vi "ADC Offset Gain_test.vi"(8 "error in (no error)":errorcluster, 9 "Sequence parameters":string[][](array[string])=[["Min limit", "Max limit", "Register sheet file", "Register Sheet"], ["", "", "CC2600.xls", "TX_BLE;Trim"], ["Reg write (addr;value)", "Operating frequency [Hz]", "", ""], ["NA", "2.44G", "", ""]], 10 "Run type":i32, 11 "Method parameters":T3={"Dev"={"Do not disturb DUT"=FALSE, "XOSC"=32000000.0, "Board type"="", "EM"="", "Configure tempboard"=TRUE, "Device specific info"=[], "Generic Object"=refnum}, "Method"={"Run type"=1, "Test name"="Current LPM2 4", "Comment"="", "Results folder"="", "AFC"=enum."Off", "Method name"="Current LPM2 4", "Method results"={"Excel brief report"=FALSE, "Spotfire report"=FALSE, "Starfish report"=FALSE}, "Operator"="", "Reference time"=timestamp(0 s since 1904-01-01), "AFC delay"=0.0, "Initialization"=enum."Enabled", "MD5 Sum"="", "HW addon board"=enum."None", "AFC Regsheet"="", "AFC Regfile"=path "", "dummy"=0.0}, "Inst"={"Instr"={"PS1"={"Name"="", "GPIB address"="", "VISA session"=""}, "PS2"={"Name"="", "GPIB address"="", "VISA session"=""}, "TC1"={"Name"="", "GPIB address"="", "VISA session"=""}, "TC2"={"Name"="", "GPIB address"="", "VISA session"=""}, "SA1"={"Name"="", "GPIB address"="", "VISA session"=""}, "SA2"={"Name"="", "GPIB address"="", "VISA session"=""}, "SG1"={"Name"="", "GPIB address"="", "VISA session"=""}, "SG2"={"Name"="", "GPIB address"="", "VISA session"=""}, "SG3"={"Name"="", "GPIB address"="", "VISA session"=""}, "MI1"={"Name"="", "GPIB address"="", "VISA session"=""}, "MI2"={"Name"="", "GPIB address"="", "VISA session"=""}, "SW SA"={"Name"="", "Controller addr"=""}, "SW SG"={"Name"="", "Controller addr"=""}, "MI3"={"Name"="", "GPIB address"="", "VISA session"=""}}, "Switchbox"={"RF Path"=0, "Cal compensation"=enum."TX", "Switchbox gain mode"="", "State"=enum."TX"}, "Instr to control (i.e. SA1)"="Default", "Intrument info string"=""}, "Sequence parameters"=[["Weight", "Min Limit", "Max Limit", "Register Sheet", "", "", "", "", "", "", "", "", ""], ["Vital", "", "1", "LPM2", "", "", "", "", "", "", "", "", ""], ["Resolution", "Reg write (addr;value)", "Chip mode", "Range", "", "", "", "", "", "", "", "", ""], ["u", "NA", "", "auto", "", "", "", "", "", "", "", "", ""]], "Cond"={"Temp logged"=25.0, "VDD1_PS1_6V"=-999.0, "VDD2_PS1_25V"=-999.0, "VDD4_PS2_25V"=-999.0, "VDD3_PS2_6V"=-999.0}, "Meas config"={"X-axis inner loop index"=32000000, "Y-axis outer loop index"=32000000, "X-axis"=[], "Y-axis"=[], "X-axis array req size"=32000000, "Y-axis array req size"=32000000, "Param description"=[], "Use meas clust for reporting"=FALSE, "Parameter index (page)"=0, "X-axis name"="", "Y-axis name"=""}} {"Cond"."VDD3_PS2_6V" format="%.3f"; "Cond"."VDD4_PS2_25V" format="%.3f"; "Cond"."VDD2_PS1_25V" format="%.3f"; "Cond"."VDD1_PS1_6V" format="%.3f"; "Method"."dummy" format="%.1p"; "Method"."AFC delay" format="%.1p"; "Dev"."XOSC" format="%.3p"}) -> (0 "error out":errorcluster, 1 "End method error":T2, 2 "Short Results":string[](array[string])=["0.00", "0.00", "0.00", "0.00"], 3 "Result summary":string[][](array[string])=[["Critical", "Output Power@2405 MHz", "-3", "4", "dBm"], ["Critical", "Output Power@2410 MHz", "-3", "4", "dBm"]])   [LabVIEW 2019]
doc: "[AutoDocStart]Performs crystal accuracy measurements. Measures the offset from ideal frequency. Primarily used for tuning XOSC capacitors and verifying XOSC trims.\n\nSweeping parameters: operating frequency, OSC override value and VDDR level\n\nResults: Offset frequency in ppm[AutoDocEnd]"
uses:
  User Lib/Utilities/Cluster definitions/Method input.ctl
  User Lib/Utilities/Cluster definitions/Device specific info.ctl
  User Lib/Utilities/Controls/Automatic Frequency Compensation types.ctl
  User Lib/Utilities/Controls/Method Reports.ctl
  User Lib/Utilities/Cluster definitions/Method Initialization.ctl
  User Lib/Utilities/Controls/HW addon boards.ctl
  User Lib/Utilities/Cluster definitions/Instr clust.ctl
  User Lib/Utilities/Switchbox control/SwitchBox_State._ENUMctl.ctl
  User Lib/Utilities/Cluster definitions/End method error cluster.ctl
  User Lib/Utilities/Cluster definitions/DUT vdd control.ctl
  User Lib/Utilities/Cluster definitions/DUT VDD4.ctl
  User Lib/Utilities/Cluster definitions/DUT VDD3.ctl
  User Lib/Utilities/Cluster definitions/DUT VDD2.ctl
  User Lib/Utilities/Cluster definitions/DUT VDD1.ctl
  User Lib/Generic chip methods/Classes/Generic_EM/Chameleon/Loki/Loki.lvclass
  <vilib>/Utility/error.llb/Clear Errors.vi
  User Lib/Generic chip methods/Classes/Generic_EM/Chameleon/65nm.lvclass
  C:/Kharon/User Lib/Generic chip methods/Classes/Generic_EM/Generic_EM/Generic_EM.lvclass
  User Lib/Generic chip methods/board_to_chip_type.vi
  User Lib/Generic chip methods/Classes/Get_Class_init.vi
  User Lib/Generic chip methods/Classes/Generic_EM/Generic_EM/Generic_EM.lvclass
  <vilib>/Analysis/NI_AALPro.lvlib
panel:
  out "x/y":dbl
  in  "Tab Control":T1(tab)
  out "Output Response [All DUTs]":u32[][](array[numeric])
  out "Measure Codes":dbl[](array[numeric])
  out "intercept":dbl
  out "slope":dbl
  out "Offset Error (mV)":dbl
  out "Gain Error (LSB)":dbl
  # "°C"
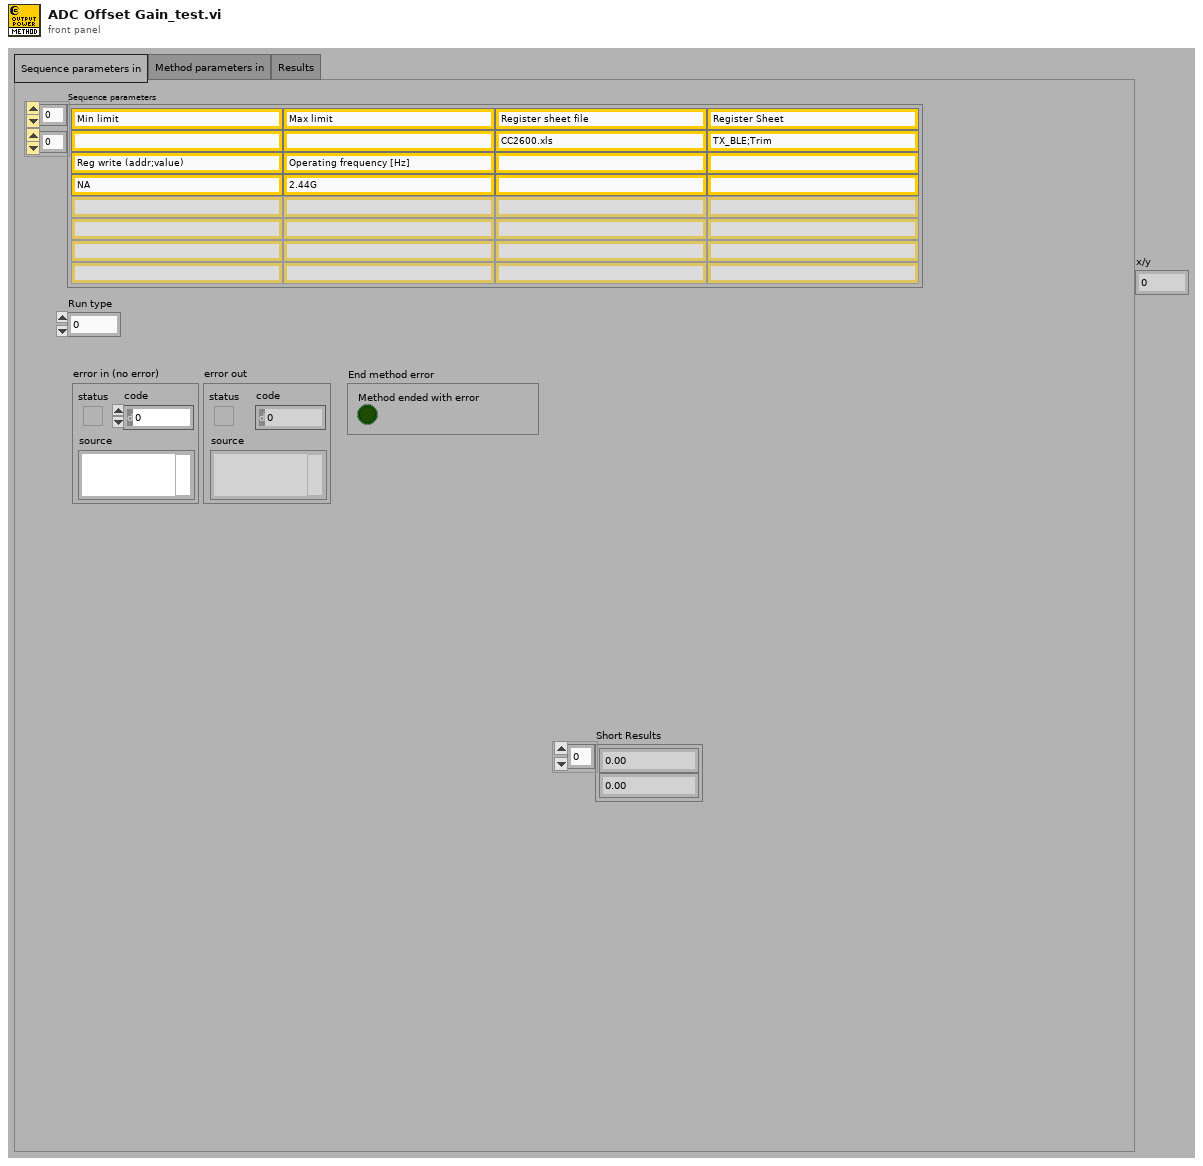
[diagram p1: front panel]
types:
  T1 = enum32{"Sequence parameters in", "Method parameters in", "Results"}
  T2 = typedef "End method error cluster.ctl" = cluster{"Method ended with error":bool}
  T3 = typedef "Method input.ctl" = cluster{"Dev":cluster{"Do not disturb DUT":bool, "XOSC":dbl, "Board type":string, "EM":string, "Configure tempboard":bool, "Device specific info":T4[], "Generic Object":refnum<class>}, "Method":cluster{"Run type":i32, "Test name":string, "Comment":string, "Results folder":string, "AFC":T5, "Method name":string, "Method results":T6, "Operator":string, "Reference time":timestamp, "AFC delay":dbl, "Initialization":T7, "MD5 Sum":string, "HW addon board":T8, "AFC Regsheet":string, "AFC Regfile":path, "dummy":dbl}, "Inst":T9, "Sequence parameters":string[][], "Cond":cluster{"Temp logged":dbl, "VDD1_PS1_6V":dbl, "VDD2_PS1_25V":dbl, "VDD4_PS2_25V":dbl, "VDD3_PS2_6V":dbl}, "Meas config":cluster{"X-axis inner loop index":i32, "Y-axis outer loop index":i32, "X-axis":string[], "Y-axis":string[], "X-axis array req size":i32, "Y-axis array req size":i32, "Param description":string[][], "Use meas clust for reporting":bool, "Parameter index (page)":i32, "X-axis name":string, "Y-axis name":string}}
  T4 = typedef "Device specific info.ctl" = cluster{"EM number":u8, "IP address":string, "Enabled":bool, "Slot no":u8, "RF path":u8, "EM name":string, "Wafer info":string, "AFC frequency ppm":dbl, "Register writes":string[][], "Meas data":string[][][], "Device comment":string}
  T5 = typedef "Automatic Frequency Compensation types.ctl" = enum16{"Off", "Compensate Instrument frequency", "Compensate DUT frequency", "Predictive - Compensate Instrument frequency", "Predictive - Compensate DUT frequency", "Do not skip re-init - Compensate Instrument frequency", "Do not skip re-init - Compensate DUT frequency"}
  T6 = typedef "Method Reports.ctl" = cluster{"Excel brief report":bool, "Spotfire report":bool, "Starfish report":bool}
  T7 = typedef "Method Initialization.ctl" = enum16{"Enabled", "Skip Instr and Device Init", "Enabled with Separate Flash", "Set PS, Device Init and Skip Instr Init", "Skip Device Init"}
  T8 = typedef "HW addon boards.ctl" = enum16{"None", "Current meas 5EM", "Stresstest 10EM"}
  T9 = typedef "Instr clust.ctl" = cluster{"Instr":cluster{"PS1":cluster{"Name":string, "GPIB address":string, "VISA session":refnum<visa-resource-name>}, "PS2":cluster{"Name":string, "GPIB address":string, "VISA session":refnum<visa-resource-name>}, "TC1":cluster{"Name":string, "GPIB address":string, "VISA session":refnum<visa-resource-name>}, "TC2":cluster{"Name":string, "GPIB address":string, "VISA session":refnum<visa-resource-name>}, "SA1":cluster{"Name":string, "GPIB address":string, "VISA session":refnum<visa-resource-name>}, "SA2":cluster{"Name":string, "GPIB address":string, "VISA session":refnum<visa-resource-name>}, "SG1":cluster{"Name":string, "GPIB address":string, "VISA session":refnum<visa-resource-name>}, "SG2":cluster{"Name":string, "GPIB address":string, "VISA session":refnum<visa-resource-name>}, "SG3":cluster{"Name":string, "GPIB address":string, "VISA session":refnum<visa-resource-name>}, "MI1":cluster{"Name":string, "GPIB address":string, "VISA session":refnum<visa-resource-name>}, "MI2":cluster{"Name":string, "GPIB address":string, "VISA session":refnum<visa-resource-name>}, "SW SA":cluster{"Name":string, "Controller addr":string}, "SW SG":cluster{"Name":string, "Controller addr":string}, "MI3":cluster{"Name":string, "GPIB address":string, "VISA session":refnum<visa-resource-name>}}, "Switchbox":cluster{"RF Path":i32, "Cal compensation":enum16{"TX", "RX", "Interferer", "No compensation", "Interferer2"}, "Switchbox gain mode":string, "State":T10}, "Instr to control (i.e. SA1)":string, "Intrument info string":string}
  T10 = typedef "SwitchBox_State._ENUMctl.ctl" = enum16{"TX", "RX", "SP:TX", "SP:RX", "SW:TX", "SW:RX"}
  T11 = typedef "DUT vdd control.ctl" = cluster{"VDD4 config":T12, "VDD3 config":T13, "VDD2 config":T14, "VDD1 config":T15}
  T12 = typedef "DUT VDD4.ctl" = u16
  T13 = typedef "DUT VDD3.ctl" = u16
  T14 = typedef "DUT VDD2.ctl" = u16
  T15 = typedef "DUT VDD1.ctl" = u16
  T16 = typedef "TFW ResponseData.ctl" = cluster{"errorCode":u32, "executionTime":u32, "processedCmdWord":u32, "responsePar":u32[], "actionCode":u32, "cmdStatus":u16}
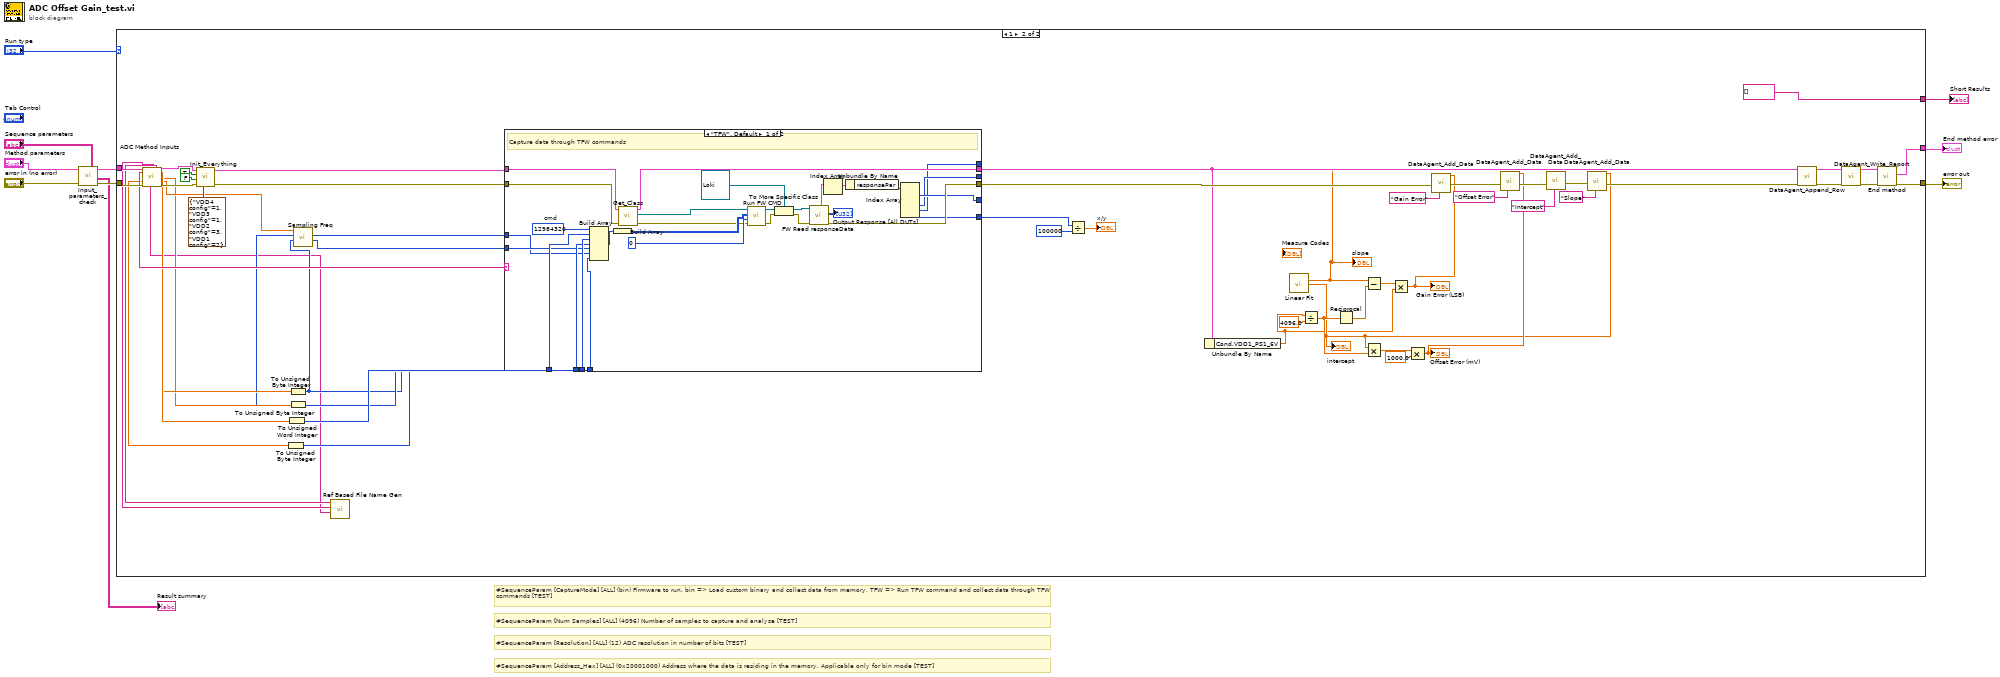
[diagram p0: block diagram]
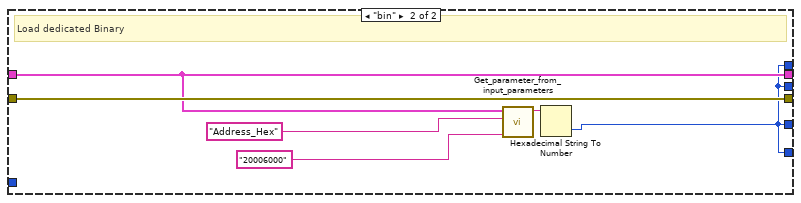
[diagram p3: hidden frame]
diagram:
  # "#SequenceParam [Num Samples] [ALL] (4096) Number of samples to capture and analyse [TEST]"
  # "#SequenceParam [CaptureMode] [ALL] (bin) Firmware to run. bin => Load custom binary and collect data from memory. TFW => Run TFW command and collect data through TFW commands [TEST]"
  # "#SequenceParam [Address_Hex] [ALL] (0x20001000) Address where the data is residing in the memory. Applicable only for bin mode [TEST]"
  # "#SequenceParam [Resolution] [ALL] (12) ADC resolution in number of bits [TEST]"
  n1 = call "Input_parameters_check.vi"("Sequence parameters"="Sequence parameters", "error in"="error in (no error)", "Method cluster in"="Method parameters") -> ("error out"=w9:errorcluster, "Result summary"=→"Result summary":string[][], "Method cluster out"=w5:T3)  [unwired: 6 in]
  n2 = case shown="1" "Run type" {
    tunnel: w9 -> [w11 w54]
    tunnel: [w11 w66] -> w10
    tunnel: w5 -> [_ w55]
    tunnel: [_ w65] -> w4
    tunnel: [_ string[] []] -> w1
    frame 0, Default {
      # "Run type 0 is only for formatting the result summary"
    }
    frame 1 {
      n3 = call "ADC Method Inputs.vi"("Method cluster in"=w55, "error in (no error)"=w54) -> ("Capture Mode"=w51:string, "ADC Channel No."=w42:dbl, "Sampling Freq String"=w38:string, "Resolution String"=w39:string, "Voltage Ref String"=w40:string, "Method cluster out"=w52:T3, "Num Samples"=w50:dbl, "Resolution"=w49:dbl, "Voltage Ref"=w47:dbl, "Sampling Freq"=w48:dbl, "error out"=w53:errorcluster)  [unwired: 6 in, 1 out]
      n4 = call "Init_Everything.vi"("VDD config"=T11 {"VDD4 config"=1, "VDD3 config"=1, "VDD2 config"=3, "VDD1 config"=2}, "error in"=w53, "Support current measurement?"=FALSE, "Override VDD Config"=TRUE, "Method cluster In"=w52) -> ("error out"=w13:errorcluster, "Method cluster out"=w14:T3)  [unwired: 3 in, 2 out]
      n5 = To Unsigned Byte Integer(number=w42) -> (unsigned 8bit integer=w43:u8)
      n6 = To Unsigned Word Integer(number=w50) -> (unsigned 16bit integer=w60:u16)
      n7 = To Unsigned Byte Integer(number=w49) -> (unsigned 8bit integer=w41:u8)
      n8 = To Unsigned Byte Integer(number=w47) -> (unsigned 8bit integer=w44:u8)
      n9 = call "Sampling Freq.vi"("Resolution"=w41, "Voltage Ref"=w44, "Sampling Freq"=w48) -> ("LGPT Count"=w46:u16, "SCOMP"=w45:u16)  [unwired: 7 in]
      n10 = call "Ref Based File Name Gen.vi"("Sampling Freq String"=w38, "Resolution String"=w39, "Voltage Ref String"=w40) -> ()  [unwired: 8 in, 1 out]
      n11 = case shown="\"TFW\", Default" w51 {
        tunnel: [w95 w97] -> w25
        tunnel: [w88 w101] -> w34
        tunnel: w13 -> [w87 w101]
        tunnel: w14 -> [w94 w97]
        tunnel: [w75 w96] -> _
        tunnel: w60 -> [w91 _]
        tunnel: w41 -> [w74 _]
        tunnel: w44 -> [w73 _]
        tunnel: w46 -> [w72 _]
        tunnel: w45 -> [w71 _]
        tunnel: w43 -> [w70 _]
        tunnel: [w69 w96] -> w16
        tunnel: [w68 w96] -> _
        tunnel: [w67 w96] -> _
        frame "TFW", Default {
          w92 = u32 12984320  # cmd
          # "Capture data through TFW commands"
          n12 = Build Array(w92, w91, w74, w73, w72, w71, w70) -> (w90:u32[])
          n13 = Build Array(w90) -> (w89:u32[][])
          n14 = call "Get_Class.vi"("error in (no error)"=w87, "Method cluster in"=w94) -> ("error out"=w85:errorcluster, "Class Out"=w84:refnum<class "Generic_EM.lvclass">, "Method cluster out"=w95:T3)  [unwired: 6 in, 1 out]
          n15 = call-dynamic "Run FW CMD.vi"("error in (no error)"=w85, "Handler"=u8 0, "cmdBuf"=w89, "Generic_EM in"=w84) -> ("error out"=w80:errorcluster, "Generic_EM out"=w83:refnum<class "Generic_EM.lvclass">)  [unwired: 6 in]
          n16 = To More Specific Class(target class=refnum<class "Loki.lvclass"> refnum ("Loki in"), reference=w83, error in=w80) -> (specific class reference=w81:refnum<class "Loki.lvclass">, error out=w79:errorcluster)
          n17 = call "FW Read responseData.vi"("error in (no error)"=w79, "Loki in"=w81) -> ("error out"=w88:errorcluster, "Output Response [All DUTs]"=→"Output Response [All DUTs]":u32[][], "Response"=w77:T16[])  [unwired: 6 in, 1 out]
          n18 = Index Array(array=w77) -> (element=w78:T16)  [unwired: 1 in]
          n19 = Unbundle By Name(w78) -> ("responsePar"=w76:u32[])
          n20 = Index Array(array=w76) -> (element #1=w75:u32, element #3=w68:u32, element #4=w67:u32, element #5=w69:u32)  [unwired: 5 in, 1 out]
        }
        frame "bin" {
          # "Load dedicated Binary"
          n21 = call "Get_parameter_from_input_parameters.vi"("Default value (used if not specified on Front Panel)"="20006000", "Parameter name"="Address_Hex" ("SA_ param name"), "Method cluster (if input param empty)"=w97) -> ("value as String"=w100:string)  [unwired: 2 in, 6 out]
          n22 = Hexadecimal String To Number(string=w100) -> (number=w96:u32)  [unwired: 2 in, 1 out]
        }
      }
      n23 = Divide(x=w16, y=u32 100000) -> (x/y=→"x/y":dbl)
      n24 = Unbundle By Name(w25) -> ("Cond.VDD1_PS1_6V"=w17:dbl)
      n25 = call <vilib>:"Linear Fit.vi"() -> ("slope"=w19:dbl, "intercept"=w18:dbl)  [unwired: 11 in, 3 out]
      "intercept" <- w18
      "slope" <- w19
      n26 = Divide(x=w17, y=4096.0) -> (x/y=w27:dbl)
      n27 = Reciprocal(x=w27) -> (1/x=w26:dbl)
      n28 = Subtract(x=w19, y=w26) -> (x-y=w28:dbl)
      n29 = Multiply(x=w18, y=w27) -> (x*y=w30:dbl)
      n30 = Multiply(x=w28, y=w17) -> (x*y=w24:dbl)
      "Gain Error (LSB)" <- w24
      n31 = Multiply(x=w30, y=1000.0) -> (x*y=w23:dbl)
      "Offset Error (mV)" <- w23
      n32 = call "DataAgent_Add_Data.vi"("ColumnName"="Gain Error", "Data"=w24, "error in (no error)"=w34) -> ("error out"=w35:errorcluster)  [unwired: 8 in]
      n33 = call "DataAgent_Add_Data.vi"("ColumnName"="Offset Error", "Data"=w23, "error in (no error)"=w35) -> ("error out"=w36:errorcluster)  [unwired: 8 in]
      n34 = call "DataAgent_Add_Data.vi"("ColumnName"="Intercept", "Data"=w19, "error in (no error)"=w36) -> ("error out"=w22:errorcluster)  [unwired: 8 in]
      n35 = call "DataAgent_Add_Data.vi"("ColumnName"="Slope", "Data"=w18, "error in (no error)"=w22) -> ("error out"=w21:errorcluster)  [unwired: 8 in]
      n36 = call "DataAgent_Append_Row.vi"("error in (no error)"=w21, "Method cluster in"=w25) -> ("error out"=w58:errorcluster, "Method cluster out"=w59:T3)  [unwired: 8 in]
      n37 = call "DataAgent_Write_Report.vi"("error in (no error)"=w58, "Method cluster in"=w59) -> ("error out"=w63:errorcluster, "Method cluster out"=w62:T3)  [unwired: 8 in]
      n38 = call "End method.vi"("error in"=w63, "Method cluster in"=w62) -> ("error out"=w66:errorcluster, "End method error"=w65:T2)  [unwired: 7 in, 1 out]
    }
  }
  "error out" <- w10
  "End method error" <- w4
  "Short Results" <- w1
